vi "Module Type.vi"(11 "GUI Helper in":refnum<class "GUI Helper.lvclass">) -> (2 "Module Type":string)   [LabVIEW 2020, in "VolatusGUI.lvlib" / "GUI Helper.lvclass"]
uses:
  GUI Helper.lvclass
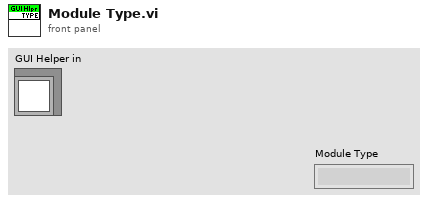
[diagram p1: front panel]
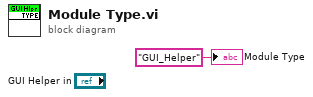
[diagram p0: block diagram]
diagram:
  "Module Type" <- "GUI_Helper" ("Module Type")
